vi "Get SHV Name.vi"(8 "error in (no error)":errorcluster, 11 "Interlock in":refnum<class "Interlock.lvclass">) -> (0 "error out":errorcluster, 2 "Name":string, 3 "Interlock out":refnum<class "Interlock.lvclass">)   [LabVIEW 2015, in "Interlocks.lvlib" / "Interlock.lvclass"]
uses:
  Interlock.lvclass
  Interlock.lvclass/Interlock.ctl
  <resource>/objmgr/ni.var.rc
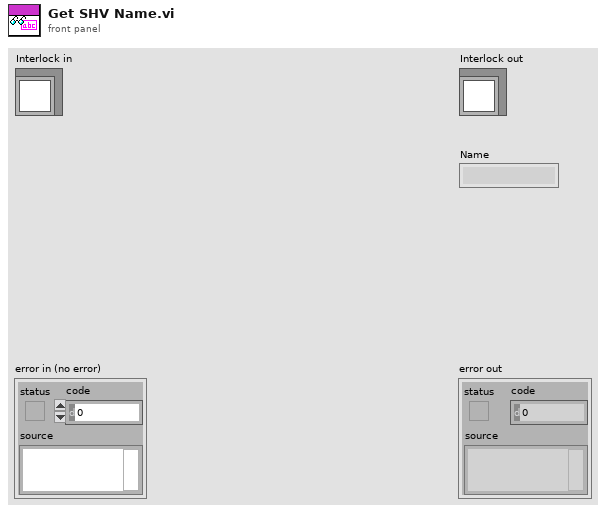
[diagram p1: front panel]
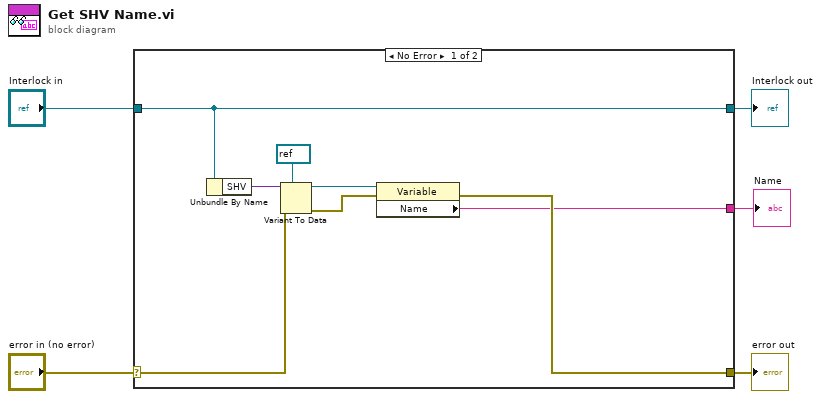
[diagram p0: block diagram]
diagram:
  n1 = case shown="No Error" "error in (no error)" {
    selector: "error in (no error)" -> [w9 w15]
    tunnel: [w11 w15] -> w4
    tunnel: [w13 w14] -> w2
    tunnel: "Interlock in" -> [w13 w14]
    tunnel: [w10 _] -> w1
    frame No Error {
      n2 = Unbundle By Name(w13) -> ("SHV"=w12:variant)
      n3 = Variant To Data(error in=w9, type=refnum<k21> refnum ("SHV"), Variant=w12) -> (data=w7:refnum<k21>, error out=w6:errorcluster)
      n4 = property class="Variable"(reference=w7, error in=w6) -> (error out=w11:errorcluster, "Name"=w10:string)  [unwired: 1 out]
    }
    frame Error {
    }
  }
  "error out" <- w4
  "Interlock out" <- w2
  "Name" <- w1
